vi "Main PC Station.vi"() -> ()   [LabVIEW 2015]
uses:
  ramki konfiguracyjne.ctl
  wyj manip.ctl
  wyj auto.ctl
  klapki.ctl
  QMH Fundamentals - Message Cluster.ctl
  CANFrameControl.ctl
  <vilib>/Utility/inputDevices.llb/closeJoystick.vi
  Gobal for ROS.vi
  <vilib>/Intelligent Energy/WebSockets API/WebSockets/WebSockets.lvlib
  <vilib>/nisyscfg/nisyscfg.lvlib
panel:
  in  "szukaj joy":bool=TRUE
  in  "wyszukaj\nxbox":bool=TRUE
  out "zakresy":cluster{"zak2":bool, "zak1":bool}
  out "Changes Require Restart":bool
  out "Detailed Result":string
  out "MANIPULATOR wy 2":T1
  in  "path":path=path "C:/Users/Kacper/Desktop/Raptorv4/LOGI PREDKOSCI/lv.csv"
  in  "LOG?":bool
  out "RAW NAPEDY":T2
  in  "ROS":bool
  in  "?":T3
  out "ROS data read":T3
  out "ERROR Prawy":dbl(graph)
  out "PIOUT Prawy":u16(graph)
  in  "ster zadane":cluster{dbl, dbl}
  in  "manual":bool
  out "stope can":bool=TRUE
  out "wyj auto":T4
  out "diody":T5
  out "przejechane ?":bool
  out "obiekt?":bool
  in  "path to JPEG file":path=path "C:/Users/Kacper/Downloads/14331560_1175035659222212_341556152_n.png"
  in  "wlacz manipulator":bool=TRUE
  out "kluster sterowan probnik":T6={"SERWO 6"=127, "SERWO 5"=127, "SERWO 4"=127, "SERWO 3"=127, "ON/OFF Wiertło"=FALSE, "Wiertło PWM"=128, "Wózek PWM"=128, "Stop głębokość"=TRUE, "Głębokość PWM"=128, "speed wózek"=0, "Wózek up"=FALSE, "Wózek down"=FALSE, "Stop wózek"=FALSE, "PROBNK ID 4"=3}
  in  "Zresetuj monitor":bool
  in  "Przestarzała data":bool
  in  "RESET STM":bool
  in  "STOP ??":bool
  in  "auto":T7={"zadany"=timestamp(0 s since 1904-01-01), "Autonomia ?"=FALSE, "Time Target (s)"=99999.0, "Reset"=FALSE, "odblokuj timer"=FALSE, "obiekt?"=FALSE, "przejechane ? "=FALSE} {"zadany" format="%<%H:%M:%S\n%x>T"}
  out "wyj pred":cluster{i16, i16, i16, i16, i16, i16} {"?" scale=-32767.0..32767.0; "?" scale=-32767.0..32767.0; "?" scale=-32767.0..32767.0; "?" scale=-32767.0..32767.0; "?" scale=-32767.0..32767.0; "?" scale=-32767.0..32767.0}
  in  "E-Stop":bool
  out "axis info":T8
  out "srednie":T9(graph)
  out "UDP connection":bool
  in  "Tab Control 2":enum32{"CAN", "FPGA H&S", "SAFETY", "Kamera"}(tab)
  in  "Tab Control":T10(tab)
  out "Digital Waveform Graph":digitalwaveform(graph)
  out "Mixed Signal Graph":T11(graph)
  in  "STM Prawy ID CAN 2":u32=1
  in  "STM Lewy ID CAN 1":u32=2
  in  "IDD PREDKOSCI 1":u8=1
  in  "IDD PREDKOSCI  2":u8=1
  in  "PRZOD L":T12={"Prąd"=20.0, "Kp"=8.0, "Ki"=3.0, "OK Button"=FALSE, "ID"=2, "IDD"=2, "Sat"=250} {"Ki" format="%.1f"; "Kp" format="%.1f"; "Prąd" format="%.1f"}
  in  "TYL L":T12={"Prąd"=20.0, "Kp"=8.0, "Ki"=3.0, "OK Button"=FALSE, "ID"=2, "IDD"=3, "Sat"=250} {"Ki" format="%.1f"; "Kp" format="%.1f"; "Prąd" format="%.1f"}
  in  "SRODEK L":T12={"Prąd"=20.0, "Kp"=8.0, "Ki"=3.0, "OK Button"=FALSE, "ID"=2, "IDD"=4, "Sat"=250} {"Ki" format="%.1f"; "Kp" format="%.1f"; "Prąd" format="%.1f"}
  in  "SRODEK P":T12={"Prąd"=20.0, "Kp"=8.0, "Ki"=3.0, "OK Button"=FALSE, "ID"=1, "IDD"=4, "Sat"=250} {"Ki" format="%.1f"; "Kp" format="%.1f"; "Prąd" format="%.1f"}
  in  "TYL P":T12={"Prąd"=20.0, "Kp"=8.0, "Ki"=3.0, "OK Button"=FALSE, "ID"=1, "IDD"=3, "Sat"=250} {"Ki" format="%.1f"; "Kp" format="%.1f"; "Prąd" format="%.1f"}
  in  "PRZOD P":T12={"Prąd"=20.0, "Kp"=8.0, "Ki"=3.0, "OK Button"=FALSE, "ID"=1, "IDD"=2, "Sat"=250} {"Ki" format="%.1f"; "Kp" format="%.1f"; "Prąd" format="%.1f"}
  in  "wagi":T13={"l przod"=1.0, "l tyl"=1.0, "l srodek"=1.0, "p przod"=1.0, "p tyl"=1.0, "p srodek"=1.0} {"l przod" format="%#.6g"}
  in  "advertise msg":string="{\"op\":\"advertise\", \"topic\":\"rio/odom\",\"type\":\"sterowanie/velocities\"}"
  in  "rosbridge port":u16=9090
  in  "rosbridge server IP":string="192.168.1.117"
  in  "STOP ROSBRIDGE":bool
  out "raw frame":string
  in  "outgoing message":T14
  in  "Topic to write":string="rio/odom"
  in  "ROSB WRITE":bool
  out "error out":errorcluster
  in  "ROSB READ":bool
  out "raw frame 2":string
  in  "stop rb":bool
  in  "Topic string":string="{ \"op\": \"subscribe\", \"topic\" : \"/cmd_to_joy\" }"
  out "error out 2":errorcluster
  in  "Wej manip":T16={"MANIPULATOR ID 3 "=3, "1 bajt"=1, "serwa i pompa"={"lewy tyl "=TRUE, "prawy tyl "=TRUE, "lewy przod "=TRUE, "środek"=TRUE, "prawy przod "=TRUE, "serwo 3"=TRUE, "serwo 4 "=TRUE, "przekaznik"=TRUE}}
  in  "ster  manual manipulator":T17 {"DRUGIE 3" scale=0.0..255.0; "PIERWSZE 2" scale=0.0..255.0; "OBROT 1" scale=0.0..255.0; "OBROT 6" scale=0.0..255.0; "CHWYTAK 5" scale=0.0..255.0; "POCHYL 4" scale=0.0..255.0}
  in  "PWM4":T12={"Prąd"=0.0, "Kp"=4.0, "Ki"=1.2, "OK Button"=FALSE, "ID"=2, "IDD"=2, "Sat"=0} {"Ki" format="%.1f"; "Kp" format="%.1f"; "Prąd" format="%.1f"}
  in  "PWM5":T12={"Prąd"=0.0, "Kp"=4.0, "Ki"=1.2, "OK Button"=FALSE, "ID"=2, "IDD"=2, "Sat"=0} {"Ki" format="%.1f"; "Kp" format="%.1f"; "Prąd" format="%.1f"}
  in  "PWM6":T12={"Prąd"=0.0, "Kp"=4.0, "Ki"=1.2, "OK Button"=FALSE, "ID"=2, "IDD"=3, "Sat"=0} {"Ki" format="%.1f"; "Kp" format="%.1f"; "Prąd" format="%.1f"}
  in  "PWM7":T12={"Prąd"=0.0, "Kp"=4.0, "Ki"=1.2000000000000002, "OK Button"=FALSE, "ID"=2, "IDD"=4, "Sat"=0} {"Ki" format="%.1f"; "Kp" format="%.1f"; "Prąd" format="%.1f"}
  in  "PWM2":T12={"Prąd"=0.0, "Kp"=4.0, "Ki"=1.2000000000000002, "OK Button"=FALSE, "ID"=1, "IDD"=3, "Sat"=0} {"Ki" format="%.1f"; "Kp" format="%.1f"; "Prąd" format="%.1f"}
  in  "PWM3":T12={"Prąd"=0.0, "Kp"=4.0, "Ki"=1.2000000000000002, "OK Button"=FALSE, "ID"=1, "IDD"=4, "Sat"=0} {"Ki" format="%.1f"; "Kp" format="%.1f"; "Prąd" format="%.1f"}
  in  "PWM1":T12={"Prąd"=0.0, "Kp"=4.0000000000000036, "Ki"=1.2000000000000002, "OK Button"=FALSE, "ID"=1, "IDD"=2, "Sat"=0} {"Ki" format="%.1f"; "Kp" format="%.1f"; "Prąd" format="%.1f"}
  in  "manual/wysylanie":bool
  out "MANIPULATOR wy":T1
  in  "pojrmniki 6":u8(slide)=127 scale=0.0..255.0
  in  "SERWO 5":u8(slide)=127 scale=0.0..255.0
  in  "SERWO 4":u8(slide)=127 scale=0.0..255.0
  in  "chwytak 3":u8(slide)=127 scale=0.0..255.0
  in  "Stop głębokość":bool
  in  "Stop wózek":bool
  in  "Wiertło PWM":u8(slide)=128 scale=0.0..255.0
  in  "Wózek PWM":u8(slide)=128 scale=0.0..255.0
  in  "Głębokość PWM":u8(slide)=128 caption="Vertical Pointer Slide" scale=0.0..255.0
  in  "ON/OFF Wiertło":bool
  in  "speed głębokość":u8
  in  "speed wózek":u8
  out "krańcówka 4":bool
  out "krańcówka 3":bool
  out "krańcówka 2":bool
  out "krańcówka":bool
  in  "PROBNK ID 4":u32=3
  in  "Wózek up":bool
  in  "Głębokość down":bool
  in  "Głębokość up":bool
  in  "Wózek down":bool
  out "glebokosc aktualna":dbl(slide) scale=-150.0..220.0
  out "wilgotność i temperatura":string
  in  "sterowanie joyem":bool
  in  "ile metrow ma przejechac ?":dbl=500.0
  out "teta":dbl
  out "Y":dbl
  out "X":dbl
  out "Location":cluster{"Y":dbl[], "Y":dbl[]}[](graph)
  in  "resset":bool
  in  "Xo":dbl
  in  "Yo":dbl
  in  "teta pocz.":dbl=90.0
  out "Yaw":dbl
  out "tekst":string
  out "po korekcie":dbl
  out "pozycje z IMU":cluster{"Yaw":dbl, "Pitch":dbl, "Roll":dbl}(graph)
  in  "laser":bool
  out "Frames":string[][](table)
  in  "Hexadecimal?":bool
  in  "Widocznosc ramek":bool=TRUE
  out "okres 100[ms]":dbl format="%.3g"
  out "ilosc mesagy":dbl
  in  "Prędkosci Prawy [4]":bool
  in  "Prędkości Lewy [5]":bool
  in  "manipulator [32]":bool
  out "przod P":cluster{"mean":dbl, i16}(graph)
  out "Środek P":cluster{"mean":dbl, i16}(graph)
  out "Tyl P":cluster{"mean":dbl, i16}(graph)
  out "TYL L 2":cluster{"mean":dbl, i16}(graph)
  out "PRZOD L 2":cluster{"mean":dbl, i16}(graph)
  out "SRODEK L 2":cluster{"mean":dbl, i16}(graph)
  out "ERROR Lewy":dbl(graph)
  out "PIOUT Lewy":i16(graph)
  in  "okres watchdoga":u32=100
  in  "wlacz watchdoga":bool
  out "temperatura":sgl(slide) scale=25.0..70.0
  in  "Total (%)":dbl(knob) scale=0.0..100.0
  in  "System Reset":bool
  out "kolejka odbior":i32
  out "kolejka wysylanie":i32
  in  "udp to sbrio":bool
  in  "eventy stop":bool
  out "send ind":i32
  in  "stop queue":bool
  out "receive ind":i32
  in  "UDP odbior in":bool
  in  "stop all":bool
  in  "UDP from sb 2":bool=TRUE
  in  "UDP to sb 2":bool=TRUE
  out "eventy ind":i32
  out "send loop":i32
  out "reciev lloop":i32
  out "safety":i32
  out "lok":i32
  out "lok1":i32
  out "jazda":i32
  out "mani":i32
  out "can":i32
  out "stope health":bool
  out "stope event":bool
  out "stope lokal":bool
  out "stope manip":bool
  out "stope jazda":bool
  out "stope lokal 2":bool
  out "stope odbior":bool
  out "stope wysyl":bool
  out "timed out?":bool
  out "wyslane\nramki":dbl
  in  "index joya\n jazda":i32
  in  "device index":i32=4
  out "zakres X":bool
  out "wysylanie":bool
  out "blokadaa":bool
  out "zakres Y":bool
  out "graph drazki":cluster{i32[], i32[]}[](graph)
  out "zakres Z":bool
  out "cluster manipulator wyswietl":T18
  out "Blokada jazda":bool
  out "graph 1":cluster{i32[], i32[]}[](graph)
  in  "max pwm skrecanie":dbl(slide)=0.5 scale=0.0..1.0
  in  "max pwm przod":dbl(slide)=0.5 min=0.0 max=255.0 scale=0.0..1.0
  out "Wysylanie jazda":bool
  # "STARE"
  # "T-"
  # "T+"
  # "gimbal 1"
  # "gimbal 2"
  # "pochyl chwytak"
  # "PWM 3 os Y\nPWM 4 os X\nPWM 5 T"
  # "chwytak O/Z"
  # "obrot chwytak"
  # "ramie 1"
  # "PWM1 os X \nPWM2 os Y\nPWM 6 T"
  # "ramie 2"
  # "obrot podstawa"
  # "Os Y+"
  # "PWM 7 T"
  # "Os X +"
  # "WYSYLANIE"
  # "- max skrecanie +"
  # "- max jazda +"
  # "hamowanie"
  # "sam OBROT"
  # "- max obrot +"
  # "OBROT"
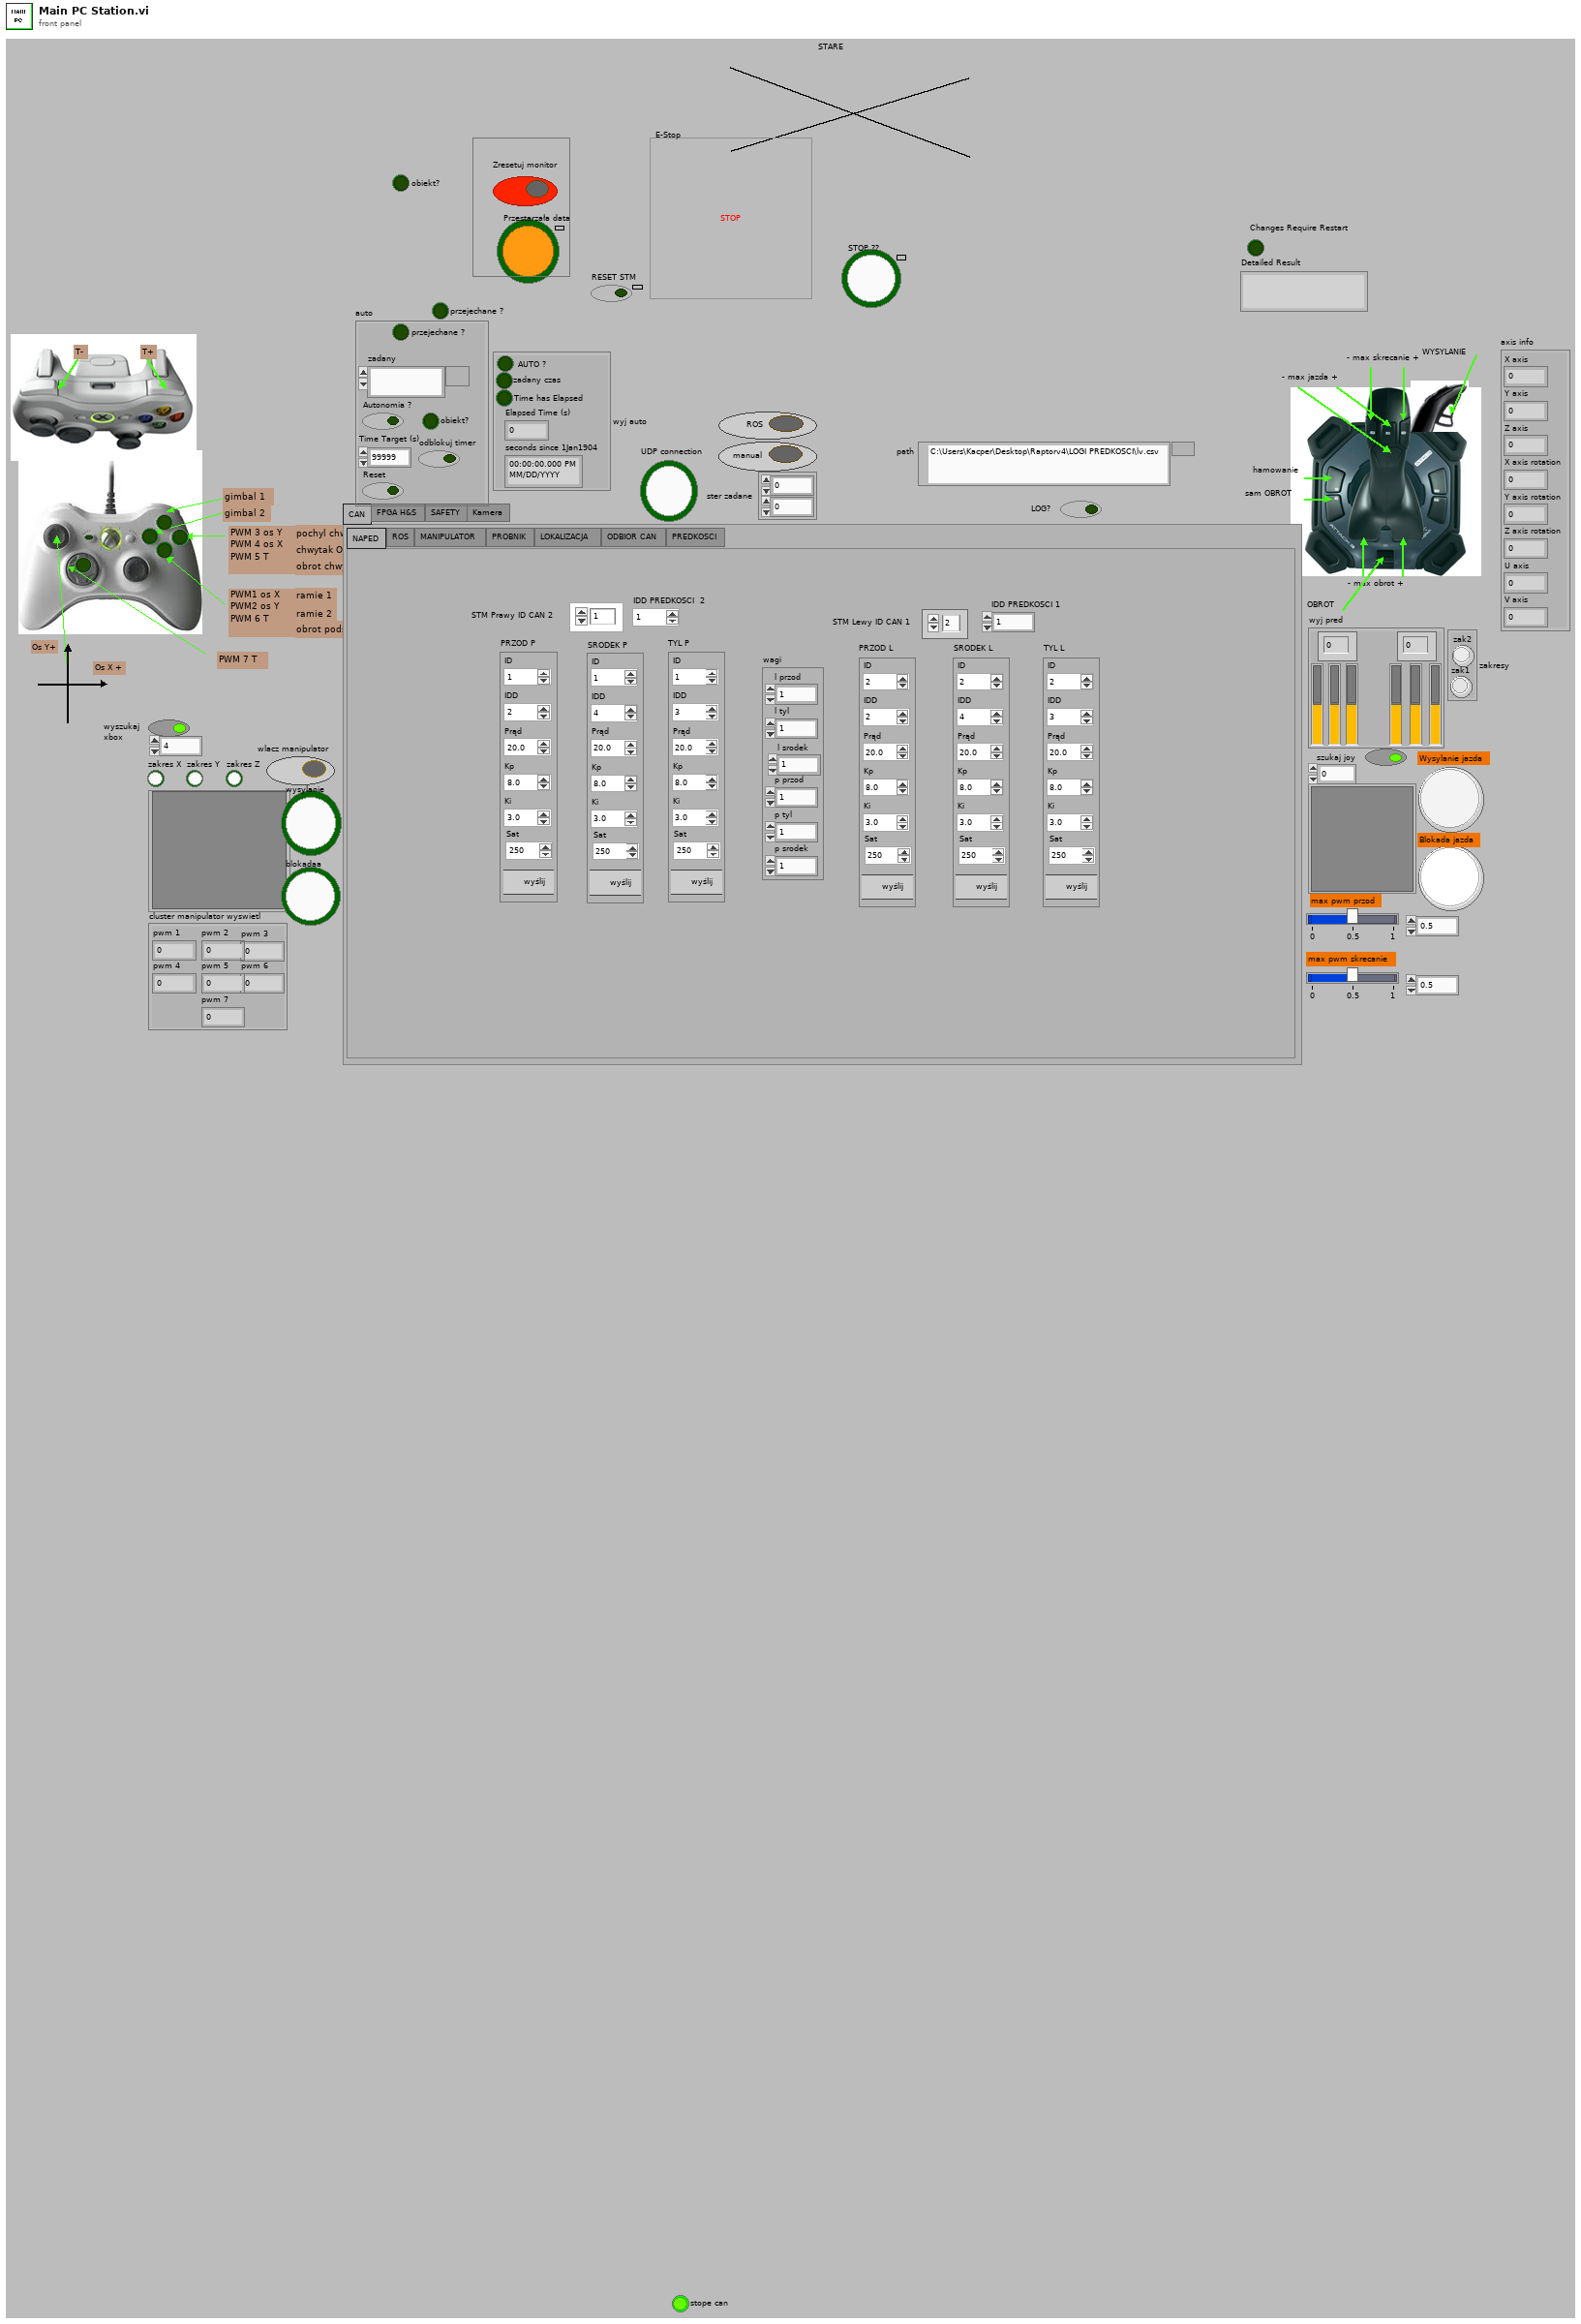
[diagram p1: front panel]
types:
  T1 = cluster{"bajt1":u8, "bajt2":u8, "bajt3":u8, "bajt4":u8, "bajt5":u8, "bajt6":u8, "bajt7":u8, "bajt8":u8}
  T2 = cluster{cluster{i16, i16, i16}, cluster{i16, i16, i16}}
  T3 = cluster{"topic":string, "msg":cluster{"header":cluster{"seq":u32, "stamp":cluster{"secs":u32, "nsecs":i32}, "frame_id":string}, "buttons":i32[], "axes":sgl[]}, "op":string}
  T4 = typedef "wyj auto.ctl" = cluster{"AUTO ?":bool, "zadany czas":bool, "Time has Elapsed":bool, "Elapsed Time (s)":dbl, "seconds since 1Jan1904":timestamp}
  T5 = typedef "wyj manip.ctl" = cluster{"button 1":bool, "button 2":bool, "button 3":bool, "button 4":bool, "button 5":bool, "POV":bool}
  T6 = cluster{"SERWO 6":u8, "SERWO 5":u8, "SERWO 4":u8, "SERWO 3":u8, "ON/OFF Wiertło":bool, "Wiertło PWM":u8, "Wózek PWM":u8, "Stop głębokość":bool, "Głębokość PWM":u8, "speed wózek":u8, "Wózek up":bool, "Wózek down":bool, "Stop wózek":bool, "PROBNK ID 4":u32}
  T7 = cluster{"zadany":timestamp, "Autonomia ?":bool, "Time Target (s)":dbl, "Reset":bool, "odblokuj timer":bool, "obiekt?":bool, "przejechane ? ":bool}
  T8 = cluster{"X axis":i32, "Y axis":i32, "Z axis":i32, "X axis rotation":i32, "Y axis rotation":i32, "Z axis rotation":i32, "U axis":i32, "V axis":i32}
  T9 = cluster{"mean":dbl, "mean":dbl, "mean":dbl, "mean":dbl, "mean":dbl, "mean":dbl}
  T10 = enum32{"NAPED", "ROS", "MANIPULATOR", "PROBNIK", "LOKALIZACJA", "ODBIOR CAN", "PREDKOSCI"}
  T11 = cluster{"digital waveform":digitalwaveform, u32[]}
  T12 = typedef "ramki konfiguracyjne.ctl" = cluster{"Prąd":dbl, "Kp":dbl, "Ki":dbl, "OK Button":bool, "ID":u32, "IDD":u8, "Sat":u8}
  T13 = cluster{"l przod":dbl, "l tyl":dbl, "l srodek":dbl, "p przod":dbl, "p tyl":dbl, "p srodek":dbl}
  T14 = cluster{"op":string, "topic":string, "msg":cluster{"vel0":i16, "vel1":i16, "vel2":i16, "vel3":i16, "vel4":i16, "vel5":i16}}
  T15 = typedef "klapki.ctl" = cluster{"lewy tyl ":bool, "prawy tyl ":bool, "lewy przod ":bool, "środek":bool, "prawy przod ":bool, "serwo 3":bool, "serwo 4 ":bool, "przekaznik":bool}
  T16 = cluster{"MANIPULATOR ID 3 ":u32, "1 bajt":u8, "serwa i pompa":T15}
  T17 = cluster{"POCHYL 4":u8, "CHWYTAK 5":u8, "OBROT 6":u8, "OBROT 1":u8, "PIERWSZE 2":u8, "DRUGIE 3":u8, "Numeric":i16}
  T18 = cluster{"pwm 1":i16, "pwm 2":i16, "pwm 3":i16, "pwm 4":i16, "pwm 5":i16, "pwm 6":i16, "pwm 7":i16}
  T19 = typedef "QMH Fundamentals - Message Cluster.ctl" = cluster{"Message":string, "Message Data":variant}
  T20 = cluster{"queue out":refnum<queue>, "error out":errorcluster}
  T21 = enum16{"Standard", "Buffered", "CRLF", "Immediate"}
  T22 = typedef "CANFrameControl.ctl" = cluster{"identifier":u32, "extended?":bool, "type":u8, "payload":u8[]}
  T23 = typedef "Wyjscia joya.ctl" = cluster{"button 1":bool, "button 2":bool, "button 3":bool, "button 4":bool, "button 5":bool, "button 6":bool, "button 7":bool, "button 8":bool, "button 9":bool, "POV":bool, "button 10":bool}
  T24 = cluster{"STM Lewy ID CAN 1":u32, "STM Prawy ID CAN 2":u32, "IDD PREDKOSCI 1":u8, "IDD PREDKOSCI  2":u8}
  T25 = cluster{"header":cluster{"seq":u32, "stamp":cluster{"secs":u32, "nsecs":i32}, "frame_id":string}, "buttons":i32[], "axes":sgl[]}
  T26 = typedef "imagedata.ctl" = cluster{"image type":i32, "image depth":i32, "image":u8[], "mask":u8[], "colors":u32[], "Rectangle":cluster{"left":i16, "top":i16, "right":i16, "bottom":i16}}
  T27 = cluster{"port wysyłania":u16, u32, "port":refnum<k16>, "error out":errorcluster}
  T28 = cluster{"Queue in":refnum<queue>, "error out":errorcluster}
  T29 = cluster{"pojrmniki 6":u8, "SERWO 5":u8, "SERWO 4":u8, "chwytak 3":u8, "ON/OFF Wiertło":bool, "Wiertło PWM":u8, "Wózek PWM":u8, "Stop głębokość":bool, "Głębokość PWM":u8, "speed wózek":u8, "Wózek up":bool, "Wózek down":bool, "Stop wózek":bool, "PROBNK ID 4":u32}
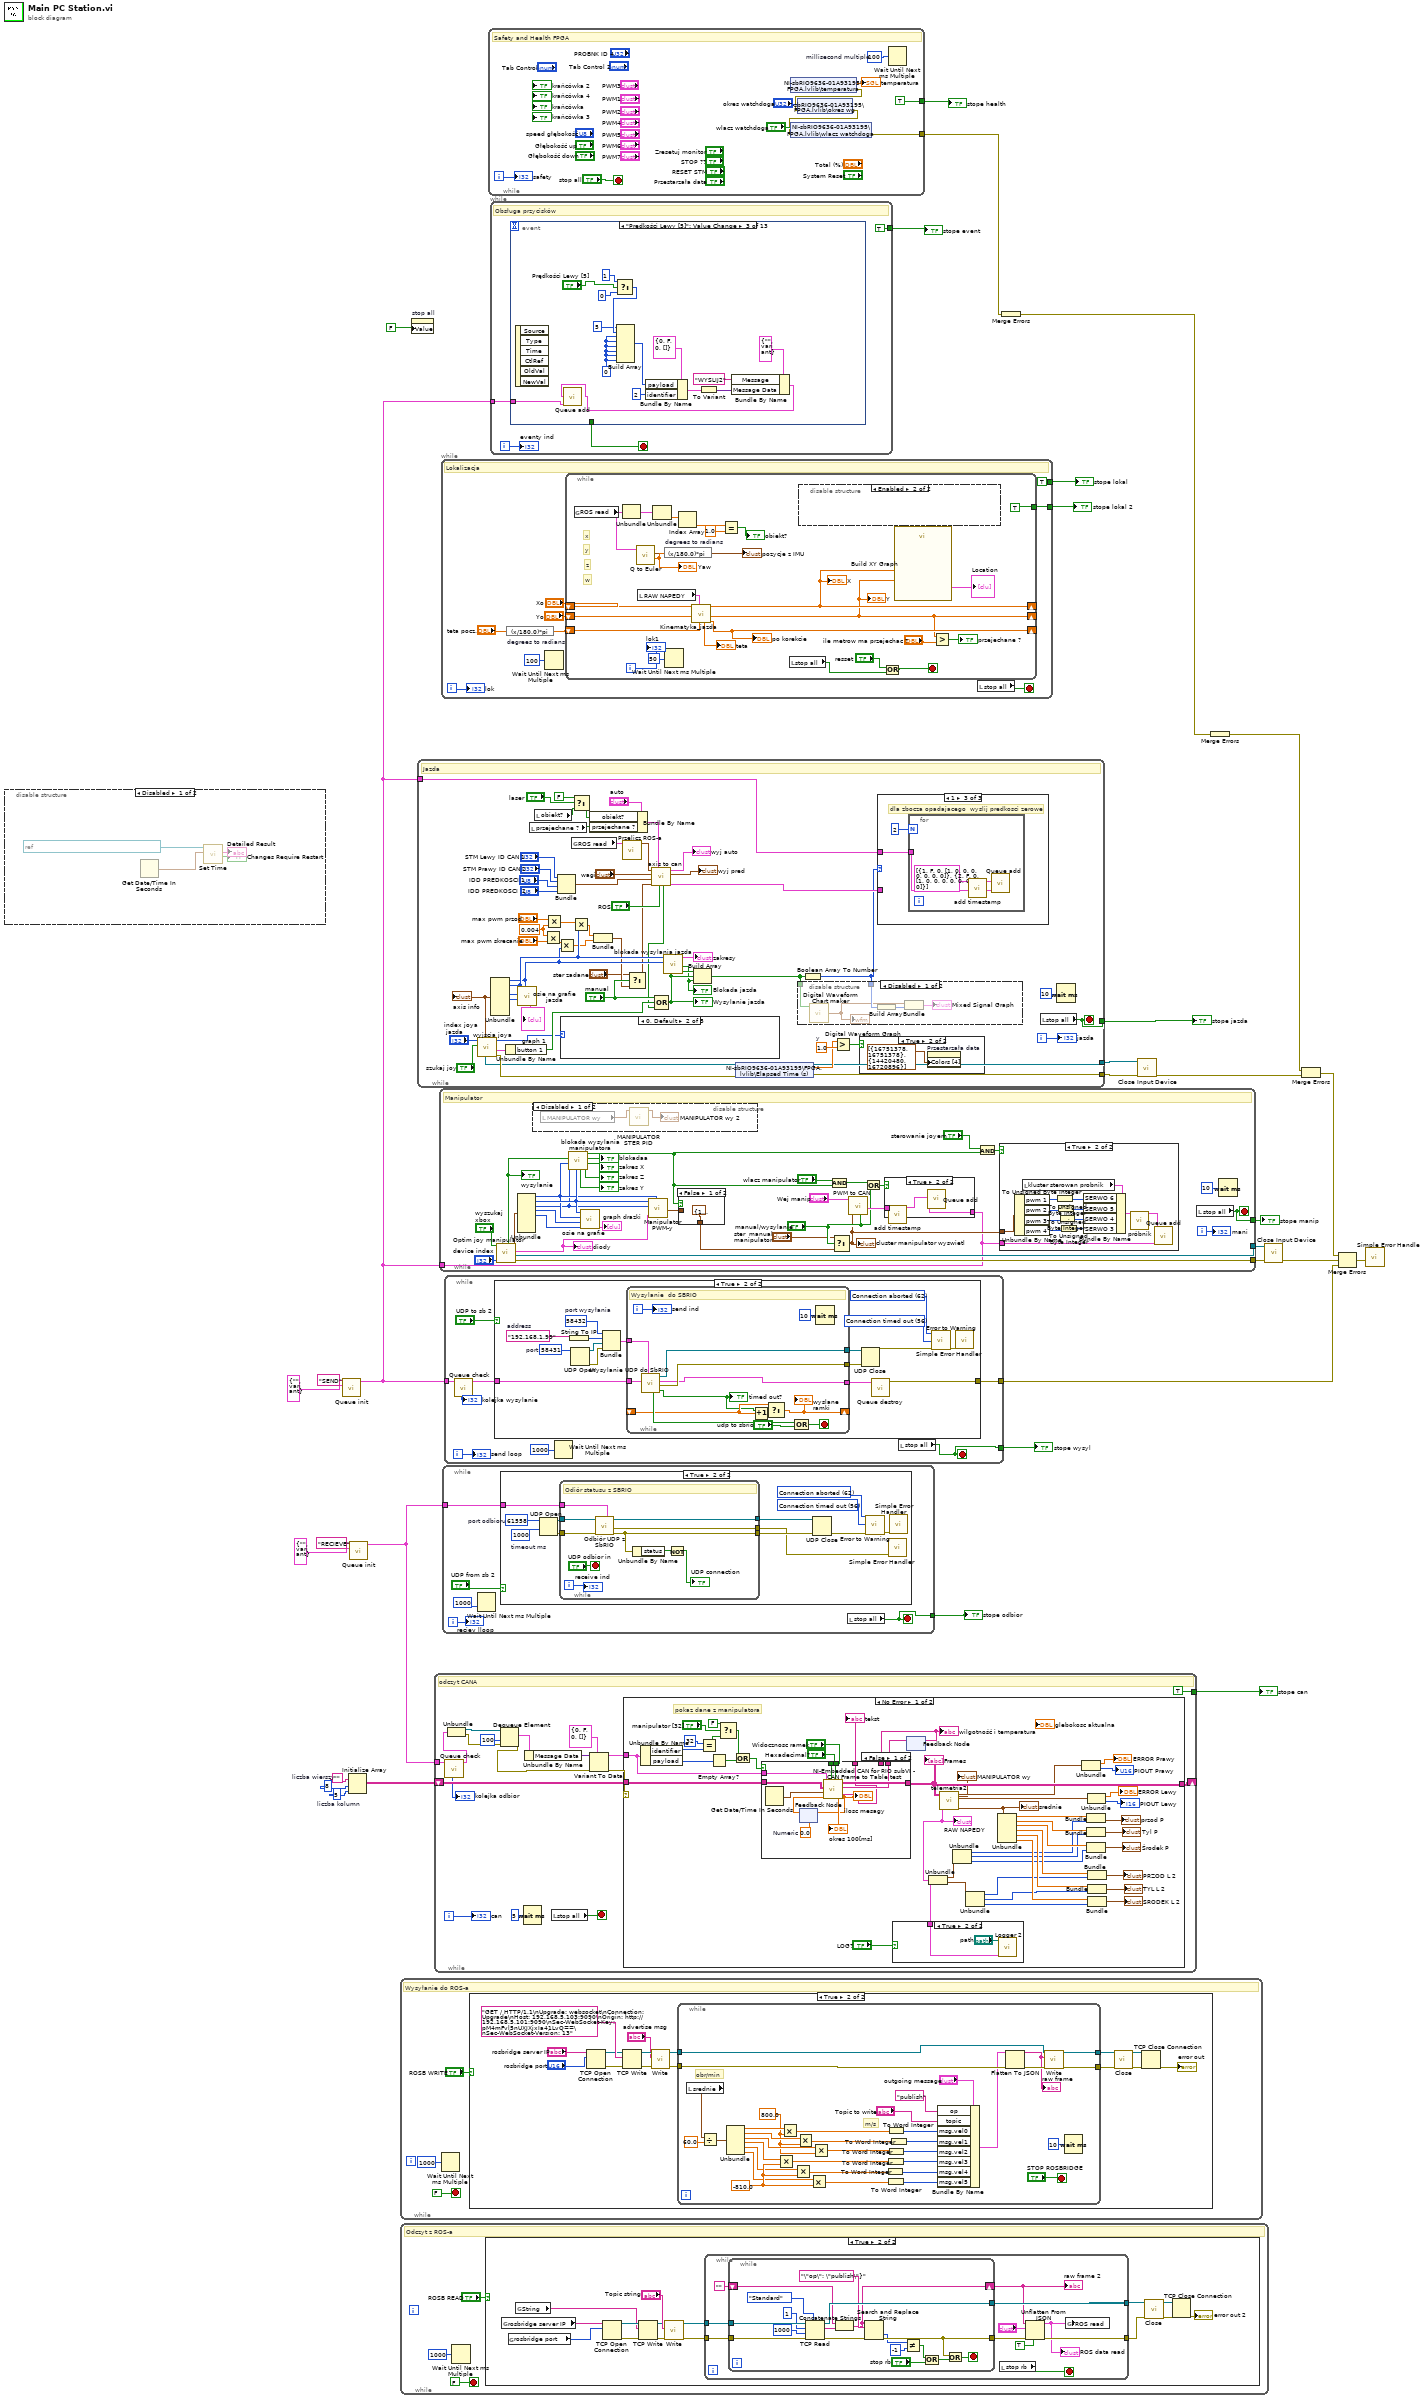
[diagram p0: block diagram]
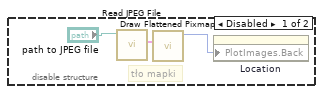
[diagram p5: hidden frame]
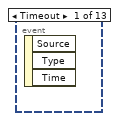
[diagram p9: hidden frame]
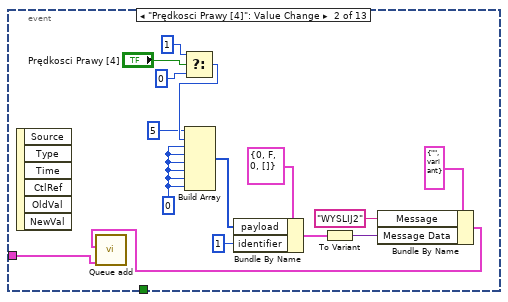
[diagram p10: hidden frame]
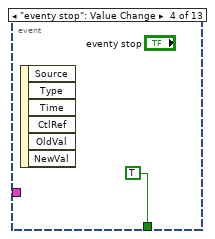
[diagram p11: hidden frame]
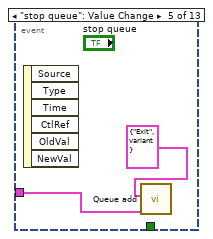
[diagram p12: hidden frame]
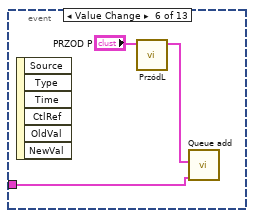
[diagram p13: hidden frame]
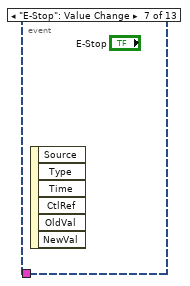
[diagram p14: hidden frame]
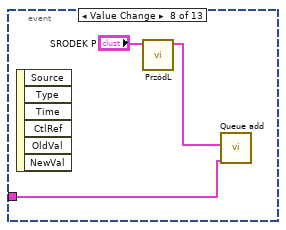
[diagram p15: hidden frame]
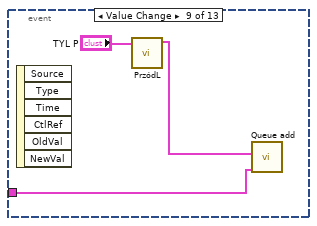
[diagram p16: hidden frame]
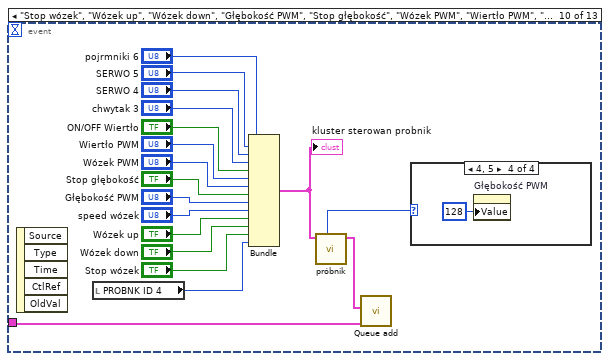
[diagram p17: hidden frame]
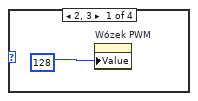
[diagram p18: hidden frame]
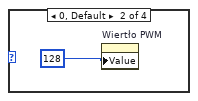
[diagram p19: hidden frame]
diagram:
  w25 = 8  # liczba wierszy
  w24 = 5  # liczba kolumn
  n1 = disable-structure shown="Disabled" {
    frame Disabled {
      n2 = Get Date/Time In Seconds() -> (seconds since 1Jan1904=w36:timestamp)
      n3 = call <vilib>:"Set Time.vi"("Time"=w36, "Session in (localhost)"=refnum<k21> "NI-sbRIO9636-01A93195 (192.168.1.99)" ("System Configuration")) -> ("Changes Require Restart"=→"Changes Require Restart":bool, "Detailed Result"=→"Detailed Result":string)  [unwired: 6 in, 2 out]
    }
    frame Enabled {
    }
  }
  n4 = call "Queue init.vi"("Message Cluster"=T19 {"Message"="", "Message Data"=variant}, "name (unnamed)"="SEND") -> ("Cluster"=w4:T20)  [unwired: 9 in]
  n5 = Initialize Array("" ("Empty String Constant"), w25, w24) -> (w22:string[][])
  n6 = call "Queue init.vi"("Message Cluster"=T19 {"Message"="", "Message Data"=variant}, "name (unnamed)"="RECIEVE") -> ("Cluster"=w1:T20)  [unwired: 9 in]
  n7 = while {
    stop <- FALSE stop-if-true
    # "Wysyłanie do ROS-a"
    n8 = Wait Until Next ms Multiple(millisecond multiple=u32 1000 ("milliseconds to wait")) -> ()  [unwired: 1 out]
    n9 = case shown="True" "ROSB WRITE" {
      frame False {
      }
      frame True {
        n10 = TCP Open Connection(address="rosbridge server IP", remote port or service name="rosbridge port") -> (connection ID=w42:refnum<k5>, error out=w44:errorcluster)  [unwired: 3 in]
        n11 = TCP Write(connection ID=w42, data in="GET / HTTP/1.1\nUpgrade: websocket\nConnection: Upgrade\nHost: 192.168.5.103:9090\nOrigin: http://192.168.5.101:9090\nSec-WebSocket-Key: pM4mFvl5nUXJXjxIa41LvQ==\nSec-WebSocket-Version: 13", error in (no error)=w44) -> (connection ID out=w53:refnum<k5>, error out=w54:errorcluster)  [unwired: 1 in, 1 out]
        n12 = call <vilib>:"Write.vi"("error in (no error)"=w54, "Data"="advertise msg", "WebSocket Connection in"=w53) -> ("error out"=w50:errorcluster, "WebSocket Connection out"=w51:refnum<k5>)  [unwired: 7 in]
        n13 = while {
          tunnel: [w87] -> w47
          tunnel: [w86] -> w48
          tunnel: w51 -> [w88]
          tunnel: w50 -> [w89]
          stop <- "STOP ROSBRIDGE" stop-if-true
          w61 = -810.0
          w62 = 800.0
          # "m/s"
          # "obr/min"
          n14 = local read "srednie"() -> (w57:T9)
          n15 = Divide(x=w57, y=60.0 ("mean")) -> (x/y=w55:T9)
          n16 = Unbundle(w55) -> ("mean"=w65:dbl, "mean"=w64:dbl, "mean"=w63:dbl, "mean"=w58:dbl, "mean"=w59:dbl, "mean"=w60:dbl)
          n17 = Multiply(x=w58, y=w61) -> (x*y=w66:dbl)
          n18 = Multiply(x=w65, y=w62) -> (x*y=w69:dbl)
          n19 = Multiply(x=w59, y=w61) -> (x*y=w67:dbl)
          n20 = Multiply(x=w64, y=w62) -> (x*y=w70:dbl)
          n21 = Multiply(x=w60, y=w61) -> (x*y=w68:dbl)
          n22 = Multiply(x=w63, y=w62) -> (x*y=w71:dbl)
          n23 = To Word Integer(number=w67) -> (16bit integer=w79:i16)
          n24 = To Word Integer(number=w66) -> (16bit integer=w80:i16)
          n25 = To Word Integer(number=w68) -> (16bit integer=w81:i16)
          n26 = To Word Integer(number=w69) -> (16bit integer=w76:i16)
          n27 = To Word Integer(number=w71) -> (16bit integer=w78:i16)
          n28 = To Word Integer(number=w70) -> (16bit integer=w77:i16)
          n29 = Bundle By Name(cluster="outgoing message", "op"="publish", "topic"="Topic to write", "msg.vel0"=w76, "msg.vel1"=w77, "msg.vel2"=w78, "msg.vel3"=w80, "msg.vel4"=w79, "msg.vel5"=w81) -> (w72:T14)
          n30 = Flatten To JSON(anything=w72, error in (no error)=w89) -> (JSON string=w83:string, 11:w85:errorcluster)  [unwired: 1 in]
          "raw frame" <- w83
          n31 = call <vilib>:"Write.vi"("error in (no error)"=w85, "Data"=w83, "WebSocket Connection in"=w88) -> ("error out"=w86:errorcluster, "WebSocket Connection out"=w87:refnum<k5>)  [unwired: 7 in]
          n32 = Wait (ms)(milliseconds to wait=u32 10) -> ()  [unwired: 1 out]
        }
        n33 = call <vilib>:"Close.vi"("error in (no error)"=w48, "WebSocket Connection in"=w47) -> ("error out"=w46:errorcluster, "WebSocket Connection in"=w45:refnum<k5>)  [unwired: 8 in]
        n34 = TCP Close Connection(connection ID=w45, error in (no error)=w46) -> (error out=→"error out":errorcluster)  [unwired: 1 in, 1 out]
      }
    }
  }
  n35 = while {
    stop <- FALSE stop-if-true
    # "Odczyt z ROS-a"
    n36 = Wait Until Next ms Multiple(millisecond multiple=u32 1000 ("milliseconds to wait")) -> ()  [unwired: 1 out]
    n37 = case shown="True" "ROSB READ" {
      frame False {
      }
      frame True {
        n38 = global read "Gobal for ROS.vi" "rosbridge server IP"() -> (w94:string)
        n39 = global read "Gobal for ROS.vi" "rosbridge port"() -> (w93:u16)
        n40 = global read "Gobal for ROS.vi" "String"() -> (w95:string)
        n41 = TCP Open Connection(address=w94, remote port or service name=w93) -> (connection ID=w107:refnum<k5>, error out=w106:errorcluster)  [unwired: 3 in]
        n42 = TCP Write(connection ID=w107, data in=w95, error in (no error)=w106) -> (connection ID out=w102:refnum<k5>, error out=w101:errorcluster)  [unwired: 1 in, 1 out]
        n43 = call <vilib>:"Write.vi"("error in (no error)"=w101, "Data"="Topic string", "WebSocket Connection in"=w102) -> ("error out"=w97:errorcluster, "WebSocket Connection out"=w98:refnum<k5>)  [unwired: 7 in]
        n44 = while {
          tunnel: [w118] -> w100
          tunnel: [w113] -> w99
          tunnel: w98 -> [w117]
          tunnel: w97 -> [w116]
          stop <- w109 stop-if-true
          n45 = while {
            tunnel: [w134] -> w118
            tunnel: [w127] -> w114
            tunnel: w117 -> [w135]
            tunnel: w116 -> [w130]
            shift-right: [w120] -> w111
            shift-left: "" -> [w122]
            stop <- w136 stop-if-true
            n46 = TCP Read(connection ID=w135, bytes to read=1, error in (no error)=w130, 7:T21."Standard" ("mode (standard)"), 9:1000 ("timeout ms (25000)")) -> (connection ID out=w134:refnum<k5>, data out=w121:string, error out=w128:errorcluster)
            n47 = Concatenate Strings(w122, w121) -> (w120:string)
            n48 = Search and Replace String(input string=w120, search string="\"op\": \"publish\"}", error in=w128) -> (offset past replacement=w124:i32, error out=w127:errorcluster)  [unwired: 5 in, 2 out]
            n49 = Not Equal?(x=w124, y=-1) -> (x != y?=w126:bool)
            n50 = Or(x=w126, y="stop rb") -> (x .or. y?=w123:bool)
            n51 = Or(x=w127, y=w123) -> (x .or. y?=w136:bool)
          }
          "raw frame 2" <- w111
          n52 = local read "stop rb"() -> (w109:bool)
          n53 = Unflatten From JSON(JSON string=w111, type and defaults="?", default null elements? (F)=TRUE, error in (no error)=w114) -> (value=w108:T3, error out=w113:errorcluster)  [unwired: 3 in]
          "ROS data read" <- w108
          n54 = global write "Gobal for ROS.vi" "ROS read"(w108) -> ()
        }
        n55 = call <vilib>:"Close.vi"("error in (no error)"=w99, "WebSocket Connection in"=w100) -> ("error out"=w103:errorcluster, "WebSocket Connection in"=w104:refnum<k5>)  [unwired: 8 in]
        n56 = TCP Close Connection(connection ID=w104, error in (no error)=w103) -> (error out=→"error out 2":errorcluster)  [unwired: 1 in, 1 out]
      }
    }
  }
  n57 = property on="stop all" class="Bool (strict)"("Value"=FALSE) -> ()  [unwired: 2 in, 2 out]
  n58 = while {
    tunnel: [w146] -> w32
    tunnel: [w176] -> w31
    tunnel: [w147] -> w18
    tunnel: w4 -> [w148]
    i -> [w160]
    stop <- w147 stop-if-true
    w155 = 0.004 ("y")
    w180 = 1.0  # y
    # "Jazda"
    n59 = call "wyjscia joya.vi"("szukaj joy"="szukaj joy", "index joya jazda"="index joya\n jazda") -> ("error out"=w177:errorcluster, "wyjscia joya"=w192:T23, "axis info"=w187:T8, "number"=w145:u32, "Refnum out"=w146:refnum<k1>)  [unwired: 3 in]
    "axis info" <- w187
    n60 = Unbundle(w187) -> ("X axis"=w167:i32, "Y axis"=w168:i32, "X axis rotation"=w189:i32, "Y axis rotation"=w190:i32)  [unwired: 4 out]
    n61 = Unbundle By Name(w192) -> ("button 1"=w191:bool)
    n62 = call "osie na grafie jazda.vi"("Y axis rotation"=w190, "X axis rotation"=w189, "Y axis"=w168, "X axis"=w167) -> ("graph 1"=→"graph 1":cluster{i32[], i32[]}[])  [unwired: 7 in]
    n63 = local read "przejechane ?"() -> (w173:bool)
    n64 = local read "obiekt?"() -> (w171:bool)
    n65 = Multiply(x=w155, y="max pwm skrecanie") -> (x*y=w158:dbl)
    n66 = Multiply(x="max pwm przod", y=w155) -> (x*y=w154:dbl)
    n67 = Bundle("STM Lewy ID CAN 1"="STM Lewy ID CAN 1", "STM Prawy ID CAN 2"="STM Prawy ID CAN 2", "IDD PREDKOSCI 1"="IDD PREDKOSCI 1", "IDD PREDKOSCI  2"="IDD PREDKOSCI  2") -> (w138:T24)  [unwired: 1 in]
    n68 = Multiply(x=w158, y=w167) -> (x*y=w159:dbl)
    n69 = case shown="0, Default" w145 {
      frame 8 {
        n70 = local read "max pwm skrecanie"() -> (w214:dbl)
        n71 = Add(x=w214, y=0.01) -> (x+y=w210:dbl)
        n72 = In Range and Coerce(upper limit=1.0, x=w210, lower limit=0.0) -> (coerced(x)=w209:dbl)  [unwired: 1 out]
        n73 = local write "max pwm skrecanie"(w209) -> ()
      }
      frame 0, Default {
      }
      frame 1 {
        n74 = local read "max pwm przod"() -> (w215:dbl)
        n75 = Add(x=w215, y=0.01) -> (x+y=w216:dbl)
        n76 = In Range and Coerce(upper limit=1.0, x=w216, lower limit=0.0) -> (coerced(x)=w217:dbl)  [unwired: 1 out]
        n77 = local write "max pwm przod"(w217) -> ()
      }
      frame 2 {
        n78 = local read "max pwm przod"() -> (w221:dbl)
        n79 = Subtract(x=w221, y=0.01) -> (x-y=w222:dbl)
        n80 = In Range and Coerce(upper limit=1.0, x=w222, lower limit=0.0) -> (coerced(x)=w223:dbl)  [unwired: 1 out]
        n81 = local write "max pwm przod"(w223) -> ()
      }
      frame 4 {
        n82 = local read "max pwm skrecanie"() -> (w232:dbl)
        n83 = Subtract(x=w232, y=0.01) -> (x-y=w229:dbl)
        n84 = In Range and Coerce(upper limit=1.0, x=w229, lower limit=0.0) -> (coerced(x)=w230:dbl)  [unwired: 1 out]
        n85 = local write "max pwm skrecanie"(w230) -> ()
      }
    }
    n86 = global read "Gobal for ROS.vi" "ROS read"() -> (w151:T3)
    n87 = Select(t=FALSE, s="laser", f=w171) -> (s? t:f=w172:bool)
    n88 = Multiply(x=w154, y=w168) -> (x*y=w181:dbl)
    n89 = Bundle By Name(cluster="auto", "obiekt?"=w172, "przejechane ?"=w173) -> (w174:T7)
    n90 = Bundle(w181, w159) -> (w152:cluster{dbl, dbl})  [unwired: 1 in]
    n91 = call "Przelicz ROS-a.vi"("ROS data"=w151) -> ("ROS data converted"=w140:cluster{dbl, dbl})  [unwired: 10 in]
    n92 = Select(t="ster zadane", s="manual", f=w152) -> (s? t:f=w139:cluster{dbl, dbl})
    n93 = call "axis to can.vi"("ROS"="ROS", "wej auto"=w174, "wej ster"=w139, "wej  ID"=w138, "wej wagi"="wagi", "ROS in"=w140) -> ("array of cans"=w188:T22[], "wyj pred"=→"wyj pred":cluster{i16, i16, i16, i16, i16, i16}, "wyj auto"=→"wyj auto":T4, "wyślij"=w141:bool)  [unwired: 2 in]
    n94 = Compound Arithmetic op=OR("manual", w191, w141) -> (w163:bool)
    "Wysylanie jazda" <- w163
    n95 = call "blokada wysylania jazda.vi"("wysylanie"=w163, "X axis"=w167, "Y axis"=w168) -> ("fall edge wysl"=w166:bool, "blokada jazdy"=w142:bool, "zakresy"=→"zakresy":cluster{"zak2":bool, "zak1":bool})  [unwired: 6 in]
    "Blokada jazda" <- w142
    n96 = Build Array(w166, w163, w142) -> (w165:bool[])
    n97 = shared-variable "NI-sbRIO9636-01A93195\\FPGA.lvlib\\Elapsed Time (s)"(error in=w177) -> (w178:dbl, error out=w176:errorcluster)
    n98 = Boolean Array To Number(Boolean array=w165) -> (number=w164:u32)
    n99 = disable-structure shown="Disabled" {
      disable-tunnel: w165 -> [w199 _]
      disable-tunnel: w164 -> [w198 _]
      frame Disabled {
        n100 = call "Digital Waveform Chart maker.vi"("Array"=w199) -> ("digital waveform"=w197:digitalwaveform)  [unwired: 3 in]
        "Digital Waveform Graph" <- w197
        n101 = Build Array(w198) -> (w196:u32[])
        n102 = Bundle("digital waveform"=w197, w196) -> (→"Mixed Signal Graph":T11)  [unwired: 1 in]
      }
      frame Enabled {
      }
    }
    n103 = Greater?(x=w178, y=w180) -> (0:w179:bool)
    n104 = case shown="True" w179 {
      frame False {
      }
      frame True {
        n105 = property on="Przestarzała data" class="Bool (strict)"("Colors [4]"=cluster{u32, u32}[] [{16751378, 16751378}, {14420480, 16720896}]) -> ()  [unwired: 2 in, 2 out]
      }
    }
    n106 = case shown="1" w164 {
      tunnel: w188 -> [_ w203 _]
      tunnel: w148 -> [_ w201 w204]
      frame 0, Default {
      }
      frame 2 {
        # "dodaj czas wysłania"
        # "normalana praca wysylaj dane"
        n107 = call "add timestamp.vi"("array of cans"=w203) -> ("Message Cluster"=w202:T19)  [unwired: 10 in]
        n108 = call "Queue add.vi"("Queue B in"=w201, "Message Cluster"=w202) -> ()  [unwired: 10 in]
      }
      frame 1 {
        # "dla zbocza opadajacego  wyslij predkosci zerowe"
        n109 = for {
          N: 2 -> [_]
          tunnel: w204 -> [w208]
          n110 = call "add timestamp.vi"("array of cans"=T22[] [{"identifier"=1, "extended?"=FALSE, "type"=0, "payload"=[1, 0, 0, 0, 0, 0, 0, 0]}, {"identifier"=2, "extended?"=FALSE, "type"=0, "payload"=[1, 0, 0, 0, 0, 0, 0, 0]}] ("zerowanie predkosci")) -> ("Message Cluster"=w206:T19)  [unwired: 10 in]
          n111 = call "Queue add.vi"("Queue B in"=w208, "Message Cluster"=w206) -> ()  [unwired: 10 in]
        }
      }
    }
    n112 = local read "stop all"() -> (w147:bool)
    n113 = Wait (ms)(milliseconds to wait=u32 10) -> ()  [unwired: 1 out]
    "jazda" <- w160
  }
  "stope jazda" <- w18
  n114 = while {
    shift-right: [w246] -> _
    shift-left: w22 -> [w249]
    tunnel: [TRUE] -> w13
    tunnel: w1 -> [w239]
    i -> [w247]
    stop <- w248 stop-if-true
    # "odczyt CANA"
    n115 = call "Queue check.vi"("output cluster"=w239) -> ("output cluster 2"=w235:T20, "# elements in queue"=→"kolejka odbior":i32)  [unwired: 9 in]
    n116 = Unbundle(w235) -> ("queue out"=w236:refnum<queue>, "error out"=w237:errorcluster)
    n117 = Dequeue Element(queue=w236, timeout in ms (-1)=100, error in (no error)=w237) -> (element=w234:T19, error out=w233:errorcluster)  [unwired: 2 out]
    n118 = Wait (ms)(milliseconds to wait=u32 5) -> ()  [unwired: 1 out]
    n119 = Unbundle By Name(w234) -> ("Message Data"=w245:variant)
    n120 = local read "stop all"() -> (w248:bool)
    n121 = Variant To Data(error in=w233, type=T22 {"identifier"=0, "extended?"=FALSE, "type"=0, "payload"=[]} ("CAN frame 3"), Variant=w245) -> (data=w243:T22, error out=w242:errorcluster)
    n122 = case shown="No Error" w242 {
      tunnel: w249 -> [w297 w314]
      tunnel: [w296 w314] -> w246
      tunnel: w243 -> [w293 _]
      frame No Error {
        # "pokaz dane z manipulatora"
        n123 = Unbundle By Name(w293) -> ("identifier"=w259:u32, "payload"=w292:u8[])
        n124 = Equal?(x=u32 32, y=w259) -> (x = y?=w253:bool)
        n125 = Empty Array?(array=w292) -> (empty?=w257:bool)
        n126 = Select(t=FALSE, s="manipulator [32]", f=w253) -> (s? t:f=w255:bool)
        n127 = Or(x=w255, y=w257) -> (x .or. y?=w256:bool)
        n128 = feedback #1() -> (w284:string)  [unwired: 1 in]
        "wilgotność i temperatura" <- w284
        n129 = case shown="False" w256 {
          tunnel: "Widocznosc ramek" -> [w309 _]
          tunnel: [w308 w313] -> w296
          tunnel: w297 -> [w307 w313]
          tunnel: "Hexadecimal?" -> [w306 _]
          tunnel: w293 -> [w302 _]
          tunnel: [w301 w312] -> w285
          tunnel: w284 -> [_ w312]
          tunnel: [w300 _] -> w283
          frame False {
            w303 = 0.0  # Numeric
            n130 = Get Date/Time In Seconds() -> (seconds since 1Jan1904=w310:timestamp)
            n131 = feedback #2(w303) -> (w304:dbl)
            n132 = call "NI-Embedded CAN for RIO subVI - CAN Frame to Table test.vi"("Boolean"=w309, "Hexadecimal?"=w306, "x"=w304, "timestamp"=w310, "Input Array"=w307, "CAN frame"=w302) -> ("Numeric"=w305:dbl, "string"=w301:string, "Output Array"=w308:string[][], "tekst"=w300:string, "okres 100"=→"okres 100[ms]":dbl)  [unwired: 1 in]
            "ilosc mesagy" <- w305
            n133 = feedback-in #2(w305) -> ()
          }
          frame True {
          }
        }
        "Frames" <- w296
        "tekst" <- w283
        n134 = feedback-in #1(w285) -> ()
        n135 = call "telemetria2.vi"("Output Array"=w296) -> ("ŚREDNIE NAPEDY"=w269:T9, "output 1000 Lewy"=w273:cluster{"ERROR":dbl, i16}, "out 100 prawy"=w270:cluster{"ERROR2":dbl, u16}, "MANIPULATOR wy"=→"MANIPULATOR wy":T1, "RAW NAPEDY"=w251:T2)  [unwired: 6 in]
        "srednie" <- w269
        "RAW NAPEDY" <- w251
        n136 = case shown="True" "LOG?" {
          tunnel: w251 -> [_ w298]
          frame False {
          }
          frame True {
            n137 = call "Logger 2.vi"("RAW NAPEDY 2"=w298, "path"="path") -> ()  [unwired: 10 in]
          }
        }
        n138 = Unbundle(w251) -> (w280:cluster{i16, i16, i16}, w268:cluster{i16, i16, i16})
        n139 = Unbundle(w280) -> (w266:i16, w265:i16, w264:i16)
        n140 = Unbundle(w268) -> (w263:i16, w262:i16, w261:i16)
        n141 = Unbundle(w269) -> ("mean"=w291:dbl, "mean"=w290:dbl, "mean"=w289:dbl, "mean"=w288:dbl, "mean"=w287:dbl, "mean"=w286:dbl)
        n142 = Unbundle(w270) -> ("ERROR2"=→"ERROR Prawy":dbl, →"PIOUT Prawy":u16)
        n143 = Bundle("mean"=w291, w266) -> (→"przod P":cluster{"mean":dbl, i16})  [unwired: 1 in]
        n144 = Bundle("mean"=w290, w265) -> (→"Tyl P":cluster{"mean":dbl, i16})  [unwired: 1 in]
        n145 = Bundle("mean"=w289, w264) -> (→"Środek P":cluster{"mean":dbl, i16})  [unwired: 1 in]
        n146 = Unbundle(w273) -> ("ERROR"=→"ERROR Lewy":dbl, →"PIOUT Lewy":i16)
        n147 = Bundle("mean"=w288, w263) -> (→"PRZOD L 2":cluster{"mean":dbl, i16})  [unwired: 1 in]
        n148 = Bundle("mean"=w287, w262) -> (→"TYL L 2":cluster{"mean":dbl, i16})  [unwired: 1 in]
        n149 = Bundle("mean"=w286, w261) -> (→"SRODEK L 2":cluster{"mean":dbl, i16})  [unwired: 1 in]
      }
      frame Error {
      }
    }
    "can" <- w247
  }
  "stope can" <- w13
  n150 = while {
    tunnel: [w331] -> w30
    tunnel: [w334] -> w29
    tunnel: [w316] -> w17
    tunnel: w4 -> [w320]
    i -> [w328]
    stop <- w316 stop-if-true
    # "Manipulator"
    n151 = call "Optim joy manipulator.vi"("device index"="device index", "wyszukaj xbox"="wyszukaj\nxbox") -> ("error out"=w334:errorcluster, "Refnum out"=w331:refnum<k1>, "output cluster"=w329:T5, "axis info"=w318:T8, "wysylanie"=w317:bool)  [unwired: 5 in]
    "wysylanie" <- w317
    "diody" <- w329
    n152 = Unbundle(w318) -> ("X axis"=w343:i32, "Y axis"=w348:i32, "Z axis"=w327:i32, "X axis rotation"=w341:i32, "Y axis rotation"=w340:i32)  [unwired: 3 out]
    n153 = disable-structure shown="Disabled" {
      frame Disabled {
        n154 = local read "MANIPULATOR wy"() -> (w349:T1)
        n155 = call "MANIPULATOR STER PID.vi"("MANIPULATOR wy 3"=w349) -> ("MANIPULATOR wy 2"=→"MANIPULATOR wy 2":T1)  [unwired: 10 in]
      }
      frame Enabled {
      }
    }
    n156 = call "blokada wysylania manipulatora.vi"("Y"=w348, "Zaxis"=w327, "X axis"=w343, "wysylanie"=w317) -> ("zakres Z"=→"zakres Z":bool, "zakres X"=→"zakres X":bool, "blokadaa"=→"blokadaa":bool, "Wyslij"=w332:bool, "zakres Y"=→"zakres Y":bool)  [unwired: 3 in]
    n157 = call "osie na grafie.vi"("Y axis rotation"=w340, "X axis rotation"=w341, "X axis"=w343, "Y axis"=w348) -> ("graph 2"=→"graph drazki":cluster{i32[], i32[]}[])  [unwired: 7 in]
    n158 = call "Manipulator PWM-y.vi"("X axis"=w343, "output cluster"=w329, "Z axis"=w327, "Y axis"=w348) -> ("wyj pwm manip."=w335:T18)  [unwired: 7 in]
    n159 = case shown="False" w332 {
      tunnel: w335 -> [_ w368]
      tunnel: [T18 {"pwm 1"=127, "pwm 2"=127, "pwm 3"=127, "pwm 4"=127, "pwm 5"=127, "pwm 6"=127, "pwm 7"=127} ("output cluster") w368] -> w326
      frame False {
      }
      frame True {
      }
    }
    n160 = And(x="wlacz manipulator", y=w332) -> (x .and. y?=w324:bool)
    n161 = Select(t="ster  manual manipulator", s="manual/wysylanie", f=w326) -> (s? t:f=w321:T18)
    "cluster manipulator wyswietl" <- w321
    n162 = call "PWM to CAN.vi"("s"="manual/wysylanie", "cluster manipulator 2"=w321, "Cluster"="Wej manip") -> ("array of cans"=w339:T22[])  [unwired: 6 in, 2 out]
    n163 = Or(x=w324, y="manual/wysylanie") -> (x .or. y?=w325:bool)
    n164 = case shown="True" w325 {
      tunnel: w339 -> [_ w365]
      tunnel: w320 -> [_ w366]
      frame False {
      }
      frame True {
        n165 = call "add timestamp.vi"("array of cans"=w365) -> ("Message Cluster"=w364:T19)  [unwired: 10 in]
        n166 = call "Queue add.vi"("Queue B in"=w366, "Message Cluster"=w364) -> ()  [unwired: 10 in]
      }
    }
    n167 = And(x="sterowanie joyem", y=w332) -> (x .and. y?=w337:bool)
    n168 = case shown="True" w337 {
      tunnel: w321 -> [_ w357]
      tunnel: w320 -> [_ w351]
      frame False {
      }
      frame True {
        n169 = Unbundle By Name(w357) -> ("pwm 1"=w356:i16, "pwm 2"=w355:i16, "pwm 3"=w354:i16, "pwm 4"=w353:i16)
        n170 = local read "kluster sterowan probnik"() -> (w363:T6)
        n171 = To Unsigned Byte Integer(number=w356) -> (unsigned 8bit integer=w358:u8)
        n172 = To Unsigned Byte Integer(number=w355) -> (unsigned 8bit integer=w359:u8)
        n173 = To Unsigned Byte Integer(number=w354) -> (unsigned 8bit integer=w360:u8)
        n174 = To Unsigned Byte Integer(number=w353) -> (unsigned 8bit integer=w361:u8)
        n175 = Bundle By Name(cluster=w363, "SERWO 6"=w358, "SERWO 5"=w359, "SERWO 4"=w360, "SERWO 3"=w361) -> (w362:T6)
        n176 = call "próbnik.vi"("output cluster 2"=w362) -> ("Message Cluster"=w352:T19)  [unwired: 9 in, 1 out]
        n177 = call "Queue add.vi"("Queue B in"=w351, "Message Cluster"=w352) -> ()  [unwired: 10 in]
      }
    }
    n178 = local read "stop all"() -> (w316:bool)
    n179 = Wait (ms)(milliseconds to wait=u32 10) -> ()  [unwired: 1 out]
    "mani" <- w328
  }
  "stope manip" <- w17
  n180 = while {
    tunnel: [TRUE] -> w19
    tunnel: [w369] -> w16
    i -> [w371]
    stop <- w376 stop-if-true
    # "Lokalizacja"
    n181 = expression code="(x/180.0)*pi" "degrees to radians"("teta pocz.") -> (w373:dbl)
    n182 = Wait Until Next ms Multiple(millisecond multiple=u32 100) -> ()  [unwired: 1 out]
    n183 = while {
      shift-right: [w400] -> _
      shift-left: "Xo" -> [w387]
      shift-right: [w384] -> _
      shift-left: "Yo" -> [w385]
      shift-right: [w386] -> _
      shift-left: w373 -> [w401]
      tunnel: [TRUE] -> w369
      i -> [w380]
      stop <- w383 stop-if-true
      # "w"
      # "z"
      # "y"
      # "x"
      n184 = global read "Gobal for ROS.vi" "ROS read"() -> (w395:T3)
      n185 = Unbundle(w395) -> ("msg"=w396:T25)  [unwired: 2 out]
      n186 = call "Q to Euler.vi"("value"=w395) -> ("Yaw"=w394:dbl, "Waveform Chart"=→"pozycje z IMU":cluster{"Yaw":dbl, "Pitch":dbl, "Roll":dbl})  [unwired: 3 in, 2 out]
      "Yaw" <- w394
      n187 = local read "RAW NAPEDY"() -> (w378:T2)
      n188 = Unbundle(w396) -> ("axes"=w397:sgl[])  [unwired: 2 out]
      n189 = expression code="(x/180.0)*pi" "degrees to radians"(w394) -> ()  [unwired: 1 out]
      n190 = Wait Until Next ms Multiple(millisecond multiple=u32 50) -> ()  [unwired: 1 out]
      n191 = Index Array(array=w397) -> (element=w392:sgl)  [unwired: 1 in]
      n192 = call "Kinematyka_jazda.vi"("teta in"=w401, "RAW NAPEDY 2"=w378, "Yo"=w385, "Xo"=w387) -> ("po korekcie"=w386:dbl, "Y"=w384:dbl, "X"=w400:dbl, "teta"=→"teta":dbl)  [unwired: 4 in]
      "X" <- w400
      "Y" <- w384
      "po korekcie" <- w386
      n193 = Equal?(x=w392, y=sgl 1.0) -> (x = y?=→"obiekt?":bool)
      n194 = local read "stop all"() -> (w381:bool)
      n195 = disable-structure shown="Enabled" {
        frame Disabled {
          # "tło mapki"
          n196 = call <vilib>:"Read JPEG File.vi"("path to JPEG file"="path to JPEG file") -> ("image data"=w404:T26)  [unwired: 8 in, 2 out]
          n197 = call <vilib>:"Draw Flattened Pixmap.vi"("image data"=w404) -> ("new picture"=w405:picture)  [unwired: 8 in]
          n198 = property on="Location" class="XYGraph (strict)"("PlotImages.Back"=w405) -> ()  [unwired: 2 in, 2 out]
        }
        frame Enabled {
        }
      }
      n199 = Or(x="resset", y=w381) -> (x .or. y?=w383:bool)
      n200 = call "Build XY Graph"("Y Input"=w384, "X Input"=w400) -> ("XY Graph"=→"Location":cluster{"Y":dbl[], "Y":dbl[]}[])  [unwired: 8 in, 1 out]
      n201 = Greater?(x=w384, y="ile metrow ma przejechac ?") -> (0:→"przejechane ?":bool)
      "lok1" <- w380
    }
    n202 = local read "stop all"() -> (w376:bool)
    "lok" <- w371
  }
  "stope lokal" <- w19
  "stope lokal 2" <- w16
  n203 = while {
    tunnel: [w406] -> w15
    tunnel: w1 -> [w407]
    i -> [w409]
    stop <- w406 stop-if-true
    n204 = Wait Until Next ms Multiple(millisecond multiple=u32 1000 ("milliseconds to wait")) -> ()  [unwired: 1 out]
    n205 = case shown="True" "UDP from sb 2" {
      tunnel: w407 -> [_ w411]
      frame False {
      }
      frame True {
        w421 = 1000  # timeout ms
        w418 = 56 items=["No Error", "Argument Error", "Memory Full", "Out of Zone", "End of File", "File Already Open", "Generic File IO Error", "File Not Found", "File Permission Error", "Disk Full", "Duplicate Path", "Too Many Files Open", "Not Enabled", "Resource File Not Found", "Cannot Add Resource", "Resource Not Found", "Image Not Found", "Image Memory Error", "Pen Does Not Exist", "Config Bad Type", "Config Token Not Found", "Config Parse Error", "Config Memory Error", "Bad External Code Format", "Bad External Code Offset", "External Code Not Present", "Null Window", "Destroy Window Mixup", "Null Menu", "Print Aborted", "Bad Print Record", "Print Driver Error", "Windows Error During Print", "Memory Error During Print", "Print Dialog Error", "Generic Print Error", "Invalid Device Refnum", "Device Not Found", "Device Parameter Error", "Device Unit Error", "Can't Open Device", "Device Call Aborted", "Generic Error", "Cancelled By User", "Object ID Too Low", "Object ID Too High", "Object Not In Heap", "Unknown Heap", "Bad DefProc ID", "DefProc Not In Table", "Message Out Of Range", "Null Method", "Unknown Message", "Manager Call Not Supported", "Bad address", "Connection In progress", "Connection timed out", "Connection is already in progress", "Network attribute not supported", "Network error", "Address in use", "System out of memory", "Connection aborted", "Connection refused", "Connection is not connected", "Connection is already connected", "Connection closed", "Initialize error (interapplication manager)", "Bad occurrence", "Wait on unbound occurrence handler", "Occurrence queue overflow", "Bad path", "Semaphore not signaled", "Unrecognized type (interapplication manager)"] ("3rd Error to Convert")
        w419 = 62 items=["No Error", "Argument Error", "Memory Full", "Out of Zone", "End of File", "File Already Open", "Generic File IO Error", "File Not Found", "File Permission Error", "Disk Full", "Duplicate Path", "Too Many Files Open", "Not Enabled", "Resource File Not Found", "Cannot Add Resource", "Resource Not Found", "Image Not Found", "Image Memory Error", "Pen Does Not Exist", "Config Bad Type", "Config Token Not Found", "Config Parse Error", "Config Memory Error", "Bad External Code Format", "Bad External Code Offset", "External Code Not Present", "Null Window", "Destroy Window Mixup", "Null Menu", "Print Aborted", "Bad Print Record", "Print Driver Error", "Windows Error During Print", "Memory Error During Print", "Print Dialog Error", "Generic Print Error", "Invalid Device Refnum", "Device Not Found", "Device Parameter Error", "Device Unit Error", "Can't Open Device", "Device Call Aborted", "Generic Error", "Cancelled By User", "Object ID Too Low", "Object ID Too High", "Object Not In Heap", "Unknown Heap", "Bad DefProc ID", "DefProc Not In Table", "Message Out Of Range", "Null Method", "Unknown Message", "Manager Call Not Supported", "Bad address", "Connection In progress", "Connection timed out", "Connection is already in progress", "Network attribute not supported", "Network error", "Address in use", "System out of memory", "Connection aborted", "Connection refused", "Connection is not connected", "Connection is already connected", "Connection closed", "Initialize error (interapplication manager)", "Bad occurrence", "Wait on unbound occurrence handler", "Occurrence queue overflow", "Bad path", "Semaphore not signaled", "Unrecognized type (interapplication manager)"] ("1st Error to Convert")
        w413 = u16 61558  # port odbioru
        n206 = UDP Open(9:w421, 11:w413) -> (port=w414:refnum<k16>, 0:w415:errorcluster)  [unwired: 3 in, 1 out]
        n207 = while {
          tunnel: w414 -> [w427]
          tunnel: w415 -> [w428]
          tunnel: [w425] -> w416
          tunnel: [w424] -> w422
          tunnel: [w426] -> w412
          tunnel: w411 -> [w423]
          i -> [w430]
          stop <- "UDP odbior in" stop-if-true
          # "Odiór statusu z SBRIO"
          n208 = call "Odbiór UDP z SbRIO.vi"("Queue B in"=w423, "error in udp (no error)"=w428, "port"=w427) -> ("error out udp"=w424:errorcluster, "error out variant"=w426:errorcluster, "UDP Network Connection out"=w425:refnum<k16>)  [unwired: 6 in]
          n209 = Unbundle By Name(w424) -> ("status"=w431:bool)
          n210 = Not(x=w431) -> (.not. x?=→"UDP connection":bool)
          "receive ind" <- w430
        }
        n211 = UDP Close(connection ID=w416, 8:w422) -> (error out=w420:errorcluster)  [unwired: 1 out]
        n212 = call <vilib>:"Error to Warning.vi"("1st Error to Convert"=w419, "3rd Error to Convert"=w418, "error in"=w420) -> ("warning out"=w417:errorcluster)  [unwired: 3 in, 9 out]
        n213 = call <vilib>:"Simple Error Handler.vi"("error in (no error)"=w412) -> ()  [unwired: 1 in, 8 out]
        n214 = call <vilib>:"Simple Error Handler.vi"("error in (no error)"=w417) -> ()  [unwired: 1 in, 8 out]
      }
    }
    n215 = local read "stop all"() -> (w406:bool)
    "reciev lloop" <- w409
  }
  "stope odbior" <- w15
  n216 = while {
    tunnel: [w438] -> w26
    tunnel: [w433] -> w14
    tunnel: w4 -> [w436]
    i -> [w439]
    stop <- w433 stop-if-true
    n217 = call "Queue check.vi"("output cluster"=w436) -> ("output cluster 2"=w434:T20, "# elements in queue"=→"kolejka wysylanie":i32)  [unwired: 9 in]
    n218 = case shown="True" "UDP to sb 2" {
      tunnel: [w441 w444] -> w438
      tunnel: w434 -> [w442 w445]
      frame False {
        n219 = Unbundle By Name(w442) -> ("error out"=w441:errorcluster)
      }
      frame True {
        w448 = u16 58431  # port
        w451 = u16 58432  # port wysyłania
        w449 = "192.168.1.99"  # address
        w455 = 56 items=["No Error", "Argument Error", "Memory Full", "Out of Zone", "End of File", "File Already Open", "Generic File IO Error", "File Not Found", "File Permission Error", "Disk Full", "Duplicate Path", "Too Many Files Open", "Not Enabled", "Resource File Not Found", "Cannot Add Resource", "Resource Not Found", "Image Not Found", "Image Memory Error", "Pen Does Not Exist", "Config Bad Type", "Config Token Not Found", "Config Parse Error", "Config Memory Error", "Bad External Code Format", "Bad External Code Offset", "External Code Not Present", "Null Window", "Destroy Window Mixup", "Null Menu", "Print Aborted", "Bad Print Record", "Print Driver Error", "Windows Error During Print", "Memory Error During Print", "Print Dialog Error", "Generic Print Error", "Invalid Device Refnum", "Device Not Found", "Device Parameter Error", "Device Unit Error", "Can't Open Device", "Device Call Aborted", "Generic Error", "Cancelled By User", "Object ID Too Low", "Object ID Too High", "Object Not In Heap", "Unknown Heap", "Bad DefProc ID", "DefProc Not In Table", "Message Out Of Range", "Null Method", "Unknown Message", "Manager Call Not Supported", "Bad address", "Connection In progress", "Connection timed out", "Connection is already in progress", "Network attribute not supported", "Network error", "Address in use", "System out of memory", "Connection aborted", "Connection refused", "Connection is not connected", "Connection is already connected", "Connection closed", "Initialize error (interapplication manager)", "Bad occurrence", "Wait on unbound occurrence handler", "Occurrence queue overflow", "Bad path", "Semaphore not signaled", "Unrecognized type (interapplication manager)"] ("3rd Error to Convert")
        w456 = 62 items=["No Error", "Argument Error", "Memory Full", "Out of Zone", "End of File", "File Already Open", "Generic File IO Error", "File Not Found", "File Permission Error", "Disk Full", "Duplicate Path", "Too Many Files Open", "Not Enabled", "Resource File Not Found", "Cannot Add Resource", "Resource Not Found", "Image Not Found", "Image Memory Error", "Pen Does Not Exist", "Config Bad Type", "Config Token Not Found", "Config Parse Error", "Config Memory Error", "Bad External Code Format", "Bad External Code Offset", "External Code Not Present", "Null Window", "Destroy Window Mixup", "Null Menu", "Print Aborted", "Bad Print Record", "Print Driver Error", "Windows Error During Print", "Memory Error During Print", "Print Dialog Error", "Generic Print Error", "Invalid Device Refnum", "Device Not Found", "Device Parameter Error", "Device Unit Error", "Can't Open Device", "Device Call Aborted", "Generic Error", "Cancelled By User", "Object ID Too Low", "Object ID Too High", "Object Not In Heap", "Unknown Heap", "Bad DefProc ID", "DefProc Not In Table", "Message Out Of Range", "Null Method", "Unknown Message", "Manager Call Not Supported", "Bad address", "Connection In progress", "Connection timed out", "Connection is already in progress", "Network attribute not supported", "Network error", "Address in use", "System out of memory", "Connection aborted", "Connection refused", "Connection is not connected", "Connection is already connected", "Connection closed", "Initialize error (interapplication manager)", "Bad occurrence", "Wait on unbound occurrence handler", "Occurrence queue overflow", "Bad path", "Semaphore not signaled", "Unrecognized type (interapplication manager)"] ("1st Error to Convert")
        n220 = String To IP(1:w449) -> (0:w450:u32)
        n221 = UDP Open(11:w448) -> (port=w447:refnum<k16>, 0:w446:errorcluster)  [unwired: 4 in, 1 out]
        n222 = Bundle("port wysyłania"=w451, w450, "port"=w447, "error out"=w446) -> (w453:T27)  [unwired: 1 in]
        n223 = while {
          tunnel: [w470] -> w458
          tunnel: [w472] -> w452
          tunnel: w453 -> [w465]
          tunnel: w445 -> [w464]
          tunnel: [w460] -> w443
          shift-right: [w462] -> _
          shift-left: _ -> [w461]
          i -> [w469]
          stop <- w468 stop-if-true
          # "Wysylanie  do SBRIO"
          n224 = call "Wysylanie UDP do SbRIO.vi"("Cluster"=w465, "output cluster"=w464) -> ("timed out?"=w459:bool, "error out udp"=w470:errorcluster, "output cluster 2"=w460:T28, "connection ID out"=w472:refnum<k16>, "stop error ?"=w467:bool)  [unwired: 5 in]
          "timed out?" <- w459
          n225 = Increment(x=w461) -> (x+1=w463:dbl)
          n226 = Select(t=w461, s=w459, f=w463) -> (s? t:f=w462:dbl)
          "wyslane\nramki" <- w462
          n227 = Compound Arithmetic op=OR(w467, "udp to sbrio") -> (w468:bool)
          n228 = Wait (ms)(milliseconds to wait=u32 10) -> ()  [unwired: 1 out]
          "send ind" <- w469
        }
        n229 = UDP Close(connection ID=w452, 8:w458) -> (error out=w457:errorcluster)  [unwired: 1 out]
        n230 = call "Queue destroy.vi"("output cluster"=w443) -> ("error out"=w444:errorcluster)  [unwired: 10 in]
        n231 = call <vilib>:"Error to Warning.vi"("1st Error to Convert"=w456, "3rd Error to Convert"=w455, "error in"=w457) -> ("warning out"=w454:errorcluster)  [unwired: 3 in, 9 out]
        n232 = call <vilib>:"Simple Error Handler.vi"("error in (no error)"=w454) -> ()  [unwired: 1 in, 8 out]
      }
    }
    n233 = Wait Until Next ms Multiple(millisecond multiple=u32 1000 ("milliseconds to wait")) -> ()  [unwired: 1 out]
    n234 = local read "stop all"() -> (w433:bool)
    "send loop" <- w439
  }
  "stope wysyl" <- w14
  n235 = while {
    tunnel: [w477] -> w10
    tunnel: [TRUE] -> w21
    i -> [w474]
    stop <- "stop all" stop-if-true
    w481 = u32 100  # millisecond multiple
    # "Safety and Health FPGA"
    n236 = shared-variable "NI-sbRIO9636-01A93195\\FPGA.lvlib\\temperatura"() -> (→"temperatura":sgl, error out=w476:errorcluster)  [unwired: 1 in]
    n237 = shared-variable "NI-sbRIO9636-01A93195\\FPGA.lvlib\\okres wg"("okres watchdoga", error in=w476) -> (error out=w478:errorcluster)
    n238 = shared-variable "NI-sbRIO9636-01A93195\\FPGA.lvlib\\wlacz watchdoga"("wlacz watchdoga", error in=w478) -> (error out=w477:errorcluster)
    n239 = Wait Until Next ms Multiple(millisecond multiple=w481) -> ()  [unwired: 1 out]
    "safety" <- w474
  }
  "stope health" <- w21
  n240 = while {
    tunnel: [TRUE] -> w20
    tunnel: w4 -> [w483]
    i -> [w485]
    stop <- w486 stop-if-true
    # "Obsługa przycisków"
    n241 = event shown="[2] \"Prędkości Lewy [5]\": Value Change" {
      selector: _ -> [_ _ _ _ _ _ _ _ _ _ _ _ _]
      dyn-events: _ -> [_ _ _ _ _ _ _ _ _ _ _ _ _]
      timeout: _ -> [_ _ _ _ _ _ _ _ _ _ _ _ _]
      tunnel: [_ _ _ TRUE _ _ _ _ _ _ _ _ _] -> w486
      tunnel: w483 -> [_ w487 w502 _ w518 w520 _ w523 w526 w529 w550 w553 w556]
      event Timeout {
        n242 = event-data() -> ()  [unwired: 1 in, 3 out]
      }
      event "Prędkosci Prawy [4]": Value Change {
        w490 = u32 0 ("identifier")
        n243 = event-data() -> ()  [unwired: 1 in, 6 out]
        n244 = Select(t=u8 1 ("identifier"), s="Prędkosci Prawy [4]", f=u8 0 ("identifier")) -> (s? t:f=w492:u8)
        n245 = Build Array(u32 5 ("identifier"), w492, w490, w490, w490, w490, w490, w490) -> (w496:u32[])
        n246 = Bundle By Name(cluster=T22 {"identifier"=0, "extended?"=FALSE, "type"=0, "payload"=[]} ("CAN frame 2"), "payload"=w496, "identifier"=u32 1) -> (w501:T22)
        n247 = To Variant(anything=w501) -> (Variant=w498:variant)
        n248 = Bundle By Name(cluster=T19 {"Message"="", "Message Data"=variant} ("Message Cluster"), "Message"="WYSLIJ2", "Message Data"=w498) -> (w488:T19)
        n249 = call "Queue add.vi"("Queue B in"=w487, "Message Cluster"=w488) -> ()  [unwired: 10 in]
      }
      event "Prędkości Lewy [5]": Value Change {
        w506 = u32 0 ("identifier")
        n250 = event-data() -> ()  [unwired: 1 in, 6 out]
        n251 = Select(t=u8 1 ("identifier"), s="Prędkości Lewy [5]", f=u8 0 ("identifier")) -> (s? t:f=w508:u8)
        n252 = Build Array(u32 5 ("identifier"), w508, w506, w506, w506, w506, w506, w506) -> (w511:u32[])
        n253 = Bundle By Name(cluster=T22 {"identifier"=0, "extended?"=FALSE, "type"=0, "payload"=[]} ("CAN frame 2"), "payload"=w511, "identifier"=u32 2) -> (w516:T22)
        n254 = To Variant(anything=w516) -> (Variant=w513:variant)
        n255 = Bundle By Name(cluster=T19 {"Message"="", "Message Data"=variant} ("Message Cluster"), "Message"="WYSLIJ2", "Message Data"=w513) -> (w503:T19)
        n256 = call "Queue add.vi"("Queue B in"=w502, "Message Cluster"=w503) -> ()  [unwired: 10 in]
      }
      event "eventy stop": Value Change {
        n257 = event-data() -> ()  [unwired: 1 in, 6 out]
      }
      event "stop queue": Value Change {
        n258 = event-data() -> ()  [unwired: 1 in, 6 out]
        n259 = call "Queue add.vi"("Queue B in"=w518, "Message Cluster"=T19 {"Message"="Exit", "Message Data"=variant} ("element")) -> ()  [unwired: 10 in]
      }
      event Value Change {
        n260 = event-data() -> ()  [unwired: 1 in, 6 out]
        n261 = call "PrzódL.vi"("Konfiguracja"="PRZOD P") -> ("Message Cluster"=w521:T19)  [unwired: 10 in]
        n262 = call "Queue add.vi"("Queue B in"=w520, "Message Cluster"=w521) -> ()  [unwired: 10 in]
      }
      event "E-Stop": Value Change {
        n263 = event-data() -> ()  [unwired: 1 in, 6 out]
      }
      event Value Change {
        n264 = event-data() -> ()  [unwired: 1 in, 6 out]
        n265 = call "PrzódL.vi"("Konfiguracja"="SRODEK P") -> ("Message Cluster"=w524:T19)  [unwired: 10 in]
        n266 = call "Queue add.vi"("Queue B in"=w523, "Message Cluster"=w524) -> ()  [unwired: 10 in]
      }
      event Value Change {
        n267 = event-data() -> ()  [unwired: 1 in, 6 out]
        n268 = call "PrzódL.vi"("Konfiguracja"="TYL P") -> ("Message Cluster"=w527:T19)  [unwired: 10 in]
        n269 = call "Queue add.vi"("Queue B in"=w526, "Message Cluster"=w527) -> ()  [unwired: 10 in]
      }
      event "Stop wózek", "Wózek up", "Wózek down", "Głębokość PWM", "Stop głębokość", "Wózek PWM", "Wiertło PWM", "ON/OFF Wiertło", "SERWO 4", "SERWO 5", "pojrmniki 6", "chwytak 3": Value Change {
        n270 = event-data() -> ()  [unwired: 1 in, 5 out]
        n271 = local read "PROBNK ID 4"() -> (w542:u32)
        n272 = Bundle("pojrmniki 6"="pojrmniki 6", "SERWO 5"="SERWO 5", "SERWO 4"="SERWO 4", "chwytak 3"="chwytak 3", "ON/OFF Wiertło"="ON/OFF Wiertło", "Wiertło PWM"="Wiertło PWM", "Wózek PWM"="Wózek PWM", "Stop głębokość"="Stop głębokość", "Głębokość PWM"="Głębokość PWM", "speed wózek"="speed wózek", "Wózek up"="Wózek up", "Wózek down"="Wózek down", "Stop wózek"="Stop wózek", "PROBNK ID 4"=w542) -> (w530:T29)  [unwired: 1 in]
        "kluster sterowan probnik" <- w530
        n273 = call "próbnik.vi"("output cluster 2"=w530) -> ("Message Cluster"=w541:T19, "number stopy"=w535:u32)  [unwired: 9 in]
        n274 = call "Queue add.vi"("Queue B in"=w529, "Message Cluster"=w541) -> ()  [unwired: 10 in]
        n275 = case shown="4, 5" w535 {
          frame 2, 3 {
            n276 = property on="Wózek PWM" class="Slide (strict)"("Value"=u8 128 ("Wózek PWM")) -> ()  [unwired: 2 in, 2 out]
          }
          frame 0, Default {
            n277 = property on="Wiertło PWM" class="Slide (strict)"("Value"=u8 128 ("Wózek PWM")) -> ()  [unwired: 2 in, 2 out]
          }
          frame 1 {
          }
          frame 4, 5 {
            n278 = property on="Głębokość PWM" class="Slide (strict)"("Value"=u8 128 ("Wózek PWM")) -> ()  [unwired: 2 in, 2 out]
          }
        }
      }
      event Value Change {
        n279 = event-data() -> ()  [unwired: 1 in, 6 out]
        n280 = call "PrzódL.vi"("Konfiguracja"="PRZOD L") -> ("Message Cluster"=w551:T19)  [unwired: 10 in]
        n281 = call "Queue add.vi"("Queue B in"=w550, "Message Cluster"=w551) -> ()  [unwired: 10 in]
      }
      event Value Change {
        n282 = event-data() -> ()  [unwired: 1 in, 6 out]
        n283 = call "PrzódL.vi"("Konfiguracja"="TYL L") -> ("Message Cluster"=w554:T19)  [unwired: 10 in]
        n284 = call "Queue add.vi"("Queue B in"=w553, "Message Cluster"=w554) -> ()  [unwired: 10 in]
      }
      event Value Change {
        n285 = event-data() -> ()  [unwired: 1 in, 6 out]
        n286 = call "PrzódL.vi"("Konfiguracja"="SRODEK L") -> ("Message Cluster"=w557:T19)  [unwired: 10 in]
        n287 = call "Queue add.vi"("Queue B in"=w556, "Message Cluster"=w557) -> ()  [unwired: 10 in]
      }
    }
    "eventy ind" <- w485
  }
  "stope event" <- w20
  n288 = Merge Errors(w10) -> (w11:errorcluster)
  n289 = call-poly <vilib>:"Close Input Device.vi"("error in (no error)"=w31, "device ID"=w32) -> ("error out"=w9:errorcluster)  [unwired: 8 in]
  n290 = Merge Errors(w11) -> (w8:errorcluster)
  n291 = call-poly <vilib>:"Close Input Device.vi"("error in (no error)"=w29, "device ID"=w30) -> ("error out"=w7:errorcluster)  [unwired: 8 in]
  n292 = Merge Errors(w8, w9) -> (w6:errorcluster)
  n293 = Merge Errors(w6, w7, w26) -> (w27:errorcluster)
  n294 = call <vilib>:"Simple Error Handler.vi"("error in (no error)"=w27) -> ()  [unwired: 1 in, 8 out]
